vi "GetScanDataBuf.vi"(8 "错误输入（无错误）":errorcluster, 11 "ArraySize":u32) -> (0 "错误输出":errorcluster)   [LabVIEW 2014]
uses:
  X86Dll/ZXUTConfigMgr.dll
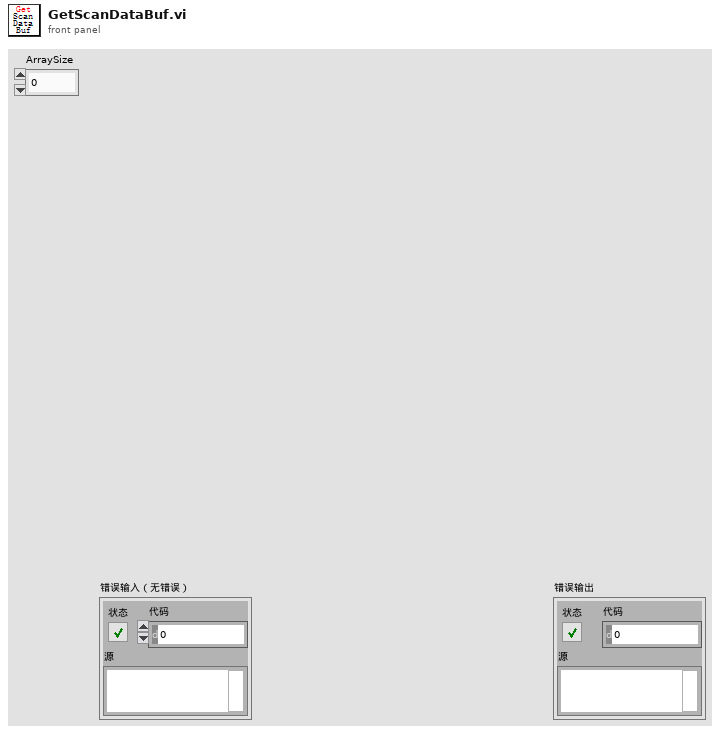
[diagram p1: front panel]
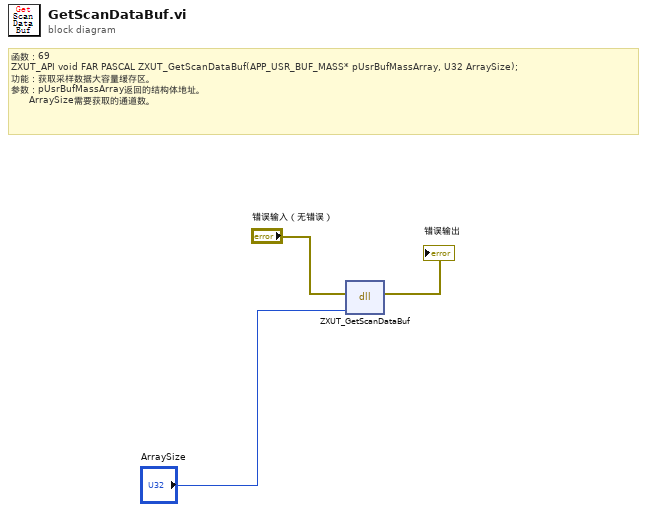
[diagram p0: block diagram]
diagram:
  # "函数：69\nZXUT_API void\tFAR PASCAL ZXUT_GetScanDataBuf(APP_USR_BUF_MASS* pUsrBufMassArray, U32 ArraySize);\n功能：获取采样数据大容量缓存区。\n参数：pUsrBufMassArray返回的结构体地址。\n      ArraySize需要获取的通道数。"
  n1 = dll-call lib="PTH2cabs F晋老师课题组在线软件合并初始化界面超声X86DllZXUTConfigMgr.dll" fn="ZXUT_GetScanDataBuf"(error in="错误输入（无错误）", "ArraySize"="ArraySize") -> (error out=→"错误输出":errorcluster)  [unwired: 4 in, 1 out]
